vi "Plugin Manager.vi"() -> ()   [LabVIEW 2016]
uses:
  Source/Engine/Classes/Plugin Manager/DSF.Engine.Runtime.Plugin Manager.lvclass
  Source/Engine/Classes/Plugin Manager/DSF.Execution.Runtime.Plugin Manager.Query Disk.Classes.vi
panel:
  out "paths":path[](array[path])
  in  "Plugins folder":path=path "C:/Users/Ryan/Desktop/Plugins"
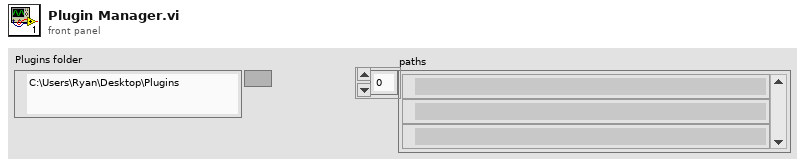
[diagram p1: front panel]
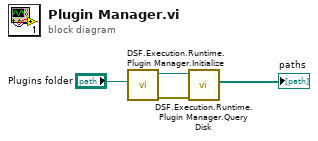
[diagram p0: block diagram]
diagram:
  n1 = call "DSF.Execution.Runtime.Plugin Manager.Initialize.vi"("Plugins folder"="Plugins folder") -> ("error out"=w2:errorcluster, "Plugin Manager out"=w3:refnum<class "DSF.Engine.Runtime.Plugin Manager.lvclass">)  [unwired: 9 in]
  n2 = call-poly "DSF.Execution.Runtime.Plugin Manager.Query Disk.vi"("error in (no error)"=w2, "Plugin Manager in"=w3) -> ("class paths"=→"paths":path[])  [unwired: 7 in, 2 out]
